vi "Read Plug-Ins Config.vi"(8 "error in (no error)":errorcluster, 10 "arguments":string[](array[string]), 11 "TestBench in":refnum<class "TestBench.lvclass">) -> (0 "error out":errorcluster, 3 "TestBench out":refnum<class "TestBench.lvclass">)   [LabVIEW 2019, in "TestBench.lvlib" / "TestBench.lvclass"]
uses:
  TestBench.lvclass
  MoldeConfiger.ctl
  TestBench.lvclass/TestBench.ctl
  Assert/Assert/Unit Test Engine Global.vi
  SignalProcessing/SignalProcessing/SignalProcessing Global.vi
  TestBench.lvlib
  SignalProcessing/SignalProcessing/SignalProcessing.lvclass
  Assert/Assert.lvlib
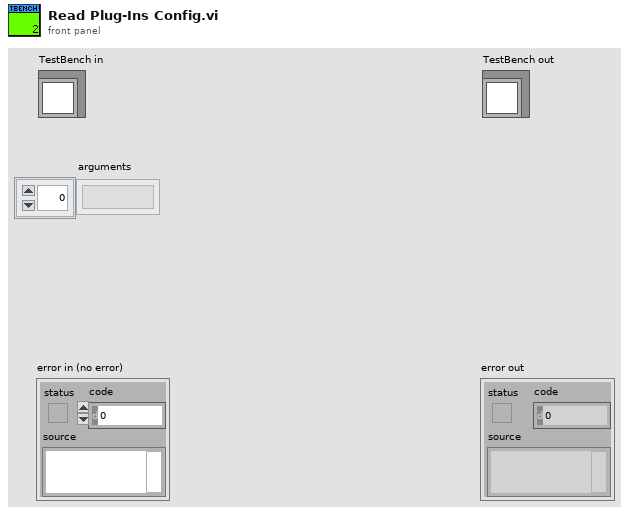
[diagram p1: front panel]
types:
  T1 = typedef "TestBench.lvlib/MoldeConfiger.ctl" = cluster{"HardwareSetupModel":string, "TestEngineModel":string, "Monitor":u16}
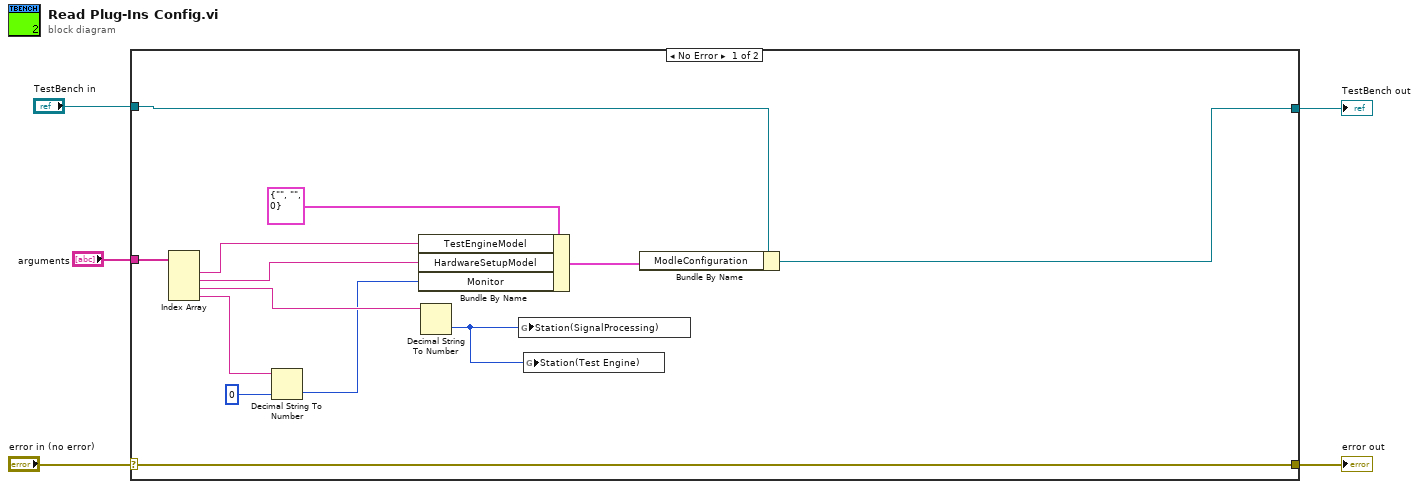
[diagram p0: block diagram]
diagram:
  n1 = case shown="No Error" "error in (no error)" {
    selector: "error in (no error)" -> [w16 w20]
    tunnel: [w16 w20] -> w4
    tunnel: [w17 w19] -> w2
    tunnel: "TestBench in" -> [w18 w19]
    tunnel: "arguments" -> [w12 _]
    frame No Error {
      n2 = Index Array(array=w12) -> (element #1=w14:string, element #2=w15:string, element #3=w10:string, element #4=w8:string)  [unwired: 4 in]
      n3 = Decimal String To Number(string=w8, default (0L)=u16 0 ("default (0 I32)")) -> (number=w6:u16)  [unwired: 1 in, 1 out]
      n4 = Bundle By Name(cluster=T1 {"HardwareSetupModel"="", "TestEngineModel"="", "Monitor"=0} ("ModleConfiguration"), "TestEngineModel"=w14, "HardwareSetupModel"=w15, "Monitor"=w6) -> (w11:T1)
      n5 = Decimal String To Number(string=w10) -> (number=w9:i32)  [unwired: 2 in, 1 out]
      n6 = global write "SignalProcessing Global.vi" "Station(SignalProcessing)"(w9) -> ()
      n7 = global write "Unit Test Engine Global.vi" "Station(Test Engine)"(w9) -> ()
      n8 = Bundle By Name(cluster=w18, "ModleConfiguration"=w11) -> (w17:refnum<class "TestBench.lvclass">)
    }
    frame Error {
    }
  }
  "error out" <- w4
  "TestBench out" <- w2
